vi "LV Exp6a.vi"   [LabVIEW 2009]
uses:
  <vilib>/NXT/Block Support/NXT_InputPort.ctl
  <vilib>/NXT/Dual Mode Library/Display/drawText.vi
  <vilib>/NXT/Dual Mode Library/Sensors/Read_Timer.vi
  <vilib>/NXT/Dual Mode Library/Sensors/Reset_Timer.vi
  <vilib>/NXT/Dual Mode Library/Waits/Wait_Num(msec).vi
panel:
  # "HiTechnic Experimenter's Kit\n\n                        Experiment 6 - Reaction Timer Variation\nThis program waits a random time, turns on the red or green LED\nand measures how much time it takes for the right button to be pressed.\n\nSee Experimenter's Kit Handbook for the SuperPro for\nmore information or go to www.hitechnic.com\n\n(c) HiTechnic 2011"
types:
  T1 = typedef "NXT_InputPort.ctl" = u8
  T2 = typedef "LVHSConnector.ctl" = cluster{"error":errorcluster, "address":string, "NXT #":i32, "Show Error":bool, "Connection":u16}
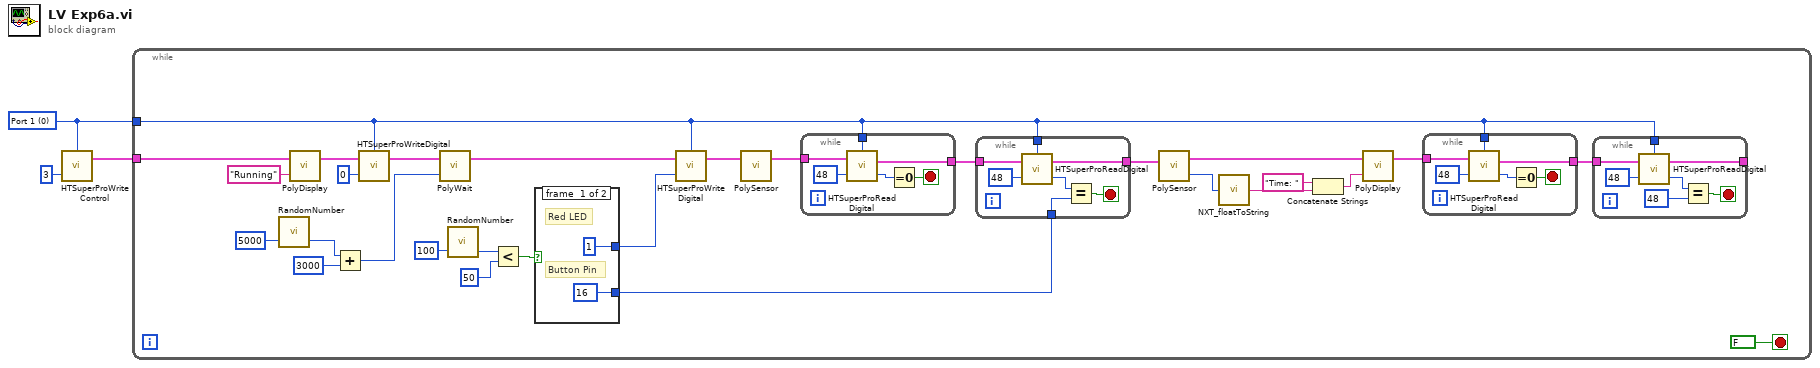
[diagram p0: block diagram]
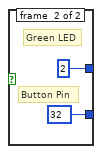
[diagram p2: hidden frame]
diagram:
  w1 = T1 0 items=["Port 1", "Port 2", "Port 3", "Port 4"] ("Port")
  n1 = call "HTSuperProWriteControl.vi"("Digital Value"=u8 3, "Port"=w1) -> ("NXT"=w2:T2)  [unwired: 3 in]
  n2 = while {
    tunnel: w2 -> [w32]
    tunnel: w1 -> [w14]
    stop <- FALSE stop-if-true
    n3 = call <vilib>:"RandomNumber.vi"("Max Value"=i16 5000) -> ("Random Number"=w27:u16)  [unwired: 2 in, 1 out]
    n4 = call-poly <vilib>:"PolyDisplay.vi"("Text"="Running", "NXT"=w32) -> ("NXT"=w30:T2)  [unwired: 2 in]
    n5 = Add(x=w27, y=i16 3000) -> (x+y=w7:u16)
    n6 = call "HTSuperProWriteDigital.vi"("Digital Value"=u8 0, "NXT"=w30, "Port"=w14) -> ("NXT"=w12:T2)  [unwired: 2 in]
    n7 = call-poly <vilib>:"PolyWait.vi"("Time (100 msec)"=w7, "NXT"=w12) -> ("NXT"=w6:T2)  [unwired: 2 in]
    n8 = call <vilib>:"RandomNumber.vi"("Max Value"=i16 100) -> ("Random Number"=w10:u16)  [unwired: 2 in, 1 out]
    n9 = Less?(x=w10, y=i16 50) -> (x < y?=w8:bool)
    n10 = case shown="True" w8 {
      tunnel: [u8 1 ("Digital Value") u8 2 ("Digital Value")] -> w5
      tunnel: [u8 16 ("Mask") u8 32 ("Mask")] -> w4
      frame #0 {
        # "Button Pin"
        # "Red LED"
      }
      frame #1 {
        # "Button Pin"
        # "Green LED"
      }
    }
    n11 = call "HTSuperProWriteDigital.vi"("Digital Value"=w5, "NXT"=w6, "Port"=w14) -> ("NXT"=w24:T2)  [unwired: 2 in]
    n12 = call-poly <vilib>:"PolySensor.vi"("NXT"=w24) -> ("NXT"=w23:T2)  [unwired: 3 in]
    n13 = while {
      tunnel: w23 -> [w62]
      tunnel: w14 -> [w58]
      tunnel: [w57] -> w25
      stop <- w59 stop-if-true
      n14 = call "HTSuperProReadDigital.vi"("Mask"=u8 48, "NXT"=w62, "Port"=w58) -> ("Digital Value"=w60:u8, "NXT"=w57:T2)  [unwired: 1 in]
      n15 = Equal To 0?(x=w60) -> (x = 0?=w59:bool)
    }
    n16 = while {
      tunnel: w25 -> [w56]
      tunnel: w14 -> [w52]
      tunnel: [w51] -> w22
      tunnel: w4 -> [w50]
      stop <- w53 stop-if-true
      n17 = call "HTSuperProReadDigital.vi"("Mask"=u8 48, "NXT"=w56, "Port"=w52) -> ("Digital Value"=w54:u8, "NXT"=w51:T2)  [unwired: 1 in]
      n18 = Equal?(x=w54, y=w50) -> (x = y?=w53:bool)
    }
    n19 = call-poly <vilib>:"PolySensor.vi"("NXT"=w22) -> ("Value (msec)"=w19:u32, "NXT"=w21:T2)  [unwired: 2 in]
    n20 = call <vilib>:"NXT_floatToString.vi"("number"=w19) -> ("string"=w18:string)
    n21 = Concatenate Strings("Time: " ("string"), w18) -> (w20:string)
    n22 = call-poly <vilib>:"PolyDisplay.vi"("Text"=w20, "NXT"=w21) -> ("NXT"=w16:T2)  [unwired: 2 in]
    n23 = while {
      tunnel: w16 -> [w49]
      tunnel: w14 -> [w45]
      tunnel: [w44] -> w15
      stop <- w46 stop-if-true
      n24 = call "HTSuperProReadDigital.vi"("Mask"=u8 48, "NXT"=w49, "Port"=w45) -> ("Digital Value"=w47:u8, "NXT"=w44:T2)  [unwired: 1 in]
      n25 = Equal To 0?(x=w47) -> (x = 0?=w46:bool)
    }
    n26 = while {
      tunnel: w15 -> [w43]
      tunnel: w14 -> [w38]
      tunnel: [w37] -> _
      stop <- w39 stop-if-true
      n27 = call "HTSuperProReadDigital.vi"("Mask"=u8 48, "NXT"=w43, "Port"=w38) -> ("Digital Value"=w41:u8, "NXT"=w37:T2)  [unwired: 1 in]
      n28 = Equal?(x=w41, y=u8 48 ("Mask")) -> (x = y?=w39:bool)
    }
  }
